vi "XIPIN_Color_Correction_Matrix_5_01_a.vi"   [LabVIEW 2017]
doc: "The Xilinx Color Correction Matrix LogiCORE can be used for color correction operations such as adjusting white balance, color cast, brightness, or contrast in an RGB image. The implementation is a 3x3 programmable coefficient matrix multiplier with offset compensation.\n------------------------------------\n<b>Need License</b> : Yes\n<b>Interface</b> : AXI4-Stream AXI4-Lite"
uses:
  <vilib>/rvi/XilinxIP/XIPIN_XNode/niFpgaXIPIN.xnode
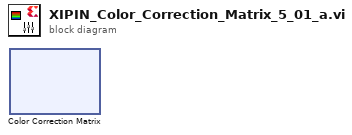
[diagram p0: block diagram]
diagram:
  n1 = xnode ("Color Correction Matrix")() -> ()
